vi "HCCTesterTimeout.vi"(11 "Timeout":dbl=5000.0) -> ()   [LabVIEW 2014]
uses:
  g_MicroZed_Interface.vi
  g_Stop.vi
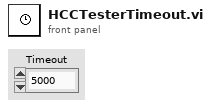
[diagram p1: front panel]
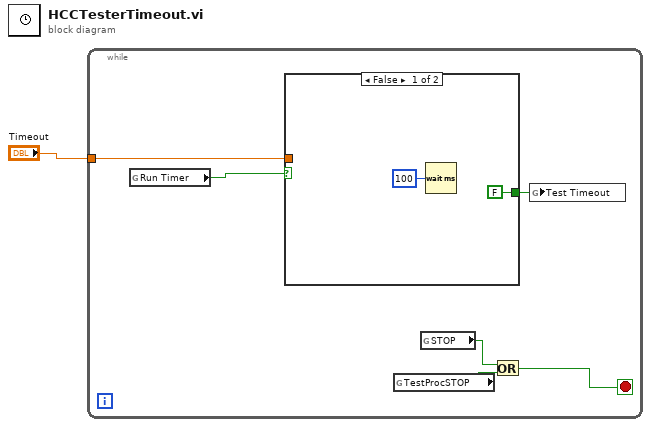
[diagram p0: block diagram]
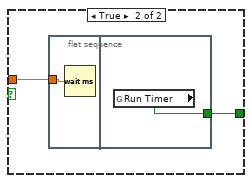
[diagram p2: hidden frame]
diagram:
  n1 = while {
    tunnel: "Timeout" -> [w7]
    stop <- w2 stop-if-true
    n2 = global read "g_MicroZed_Interface.vi" "Run Timer"() -> (w5:bool)
    n3 = case shown="False" w5 {
      tunnel: w7 -> [_ w11]
      tunnel: [FALSE w10] -> w6
      frame False {
        n4 = Wait (ms)(milliseconds to wait=u32 100) -> ()  [unwired: 1 out]
      }
      frame True {
        n5 = flat-sequence {
          tunnel: w11 -> [w12]
          tunnel: [w13] -> w10
          frame #0 {
            n6 = Wait (ms)(milliseconds to wait=w12) -> ()  [unwired: 1 out]
          }
          frame #1 {
            n7 = global read "g_MicroZed_Interface.vi" "Run Timer"() -> (w13:bool)
          }
        }
      }
    }
    n8 = global read "g_Stop.vi" "TestProcSTOP"() -> (w3:bool)
    n9 = global read "g_Stop.vi" "STOP"() -> (w4:bool)
    n10 = Or(x=w4, y=w3) -> (x .or. y?=w2:bool)
    n11 = global write "g_MicroZed_Interface.vi" "Test Timeout"(w6) -> ()
  }
